vi "GT_EncOn.vi"(2 "encoder":i16, 3 "rtn_In":cluster{"rtn":i16, "Func":string}) -> (0 "encoder out":i16, 1 "rtn_Out":cluster{"rtn":i16, "Func":string})   [LabVIEW 2014]
uses:
  VC6/gts.dll
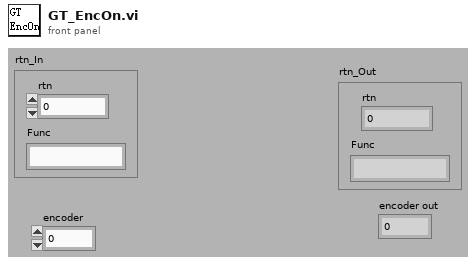
[diagram p1: front panel]
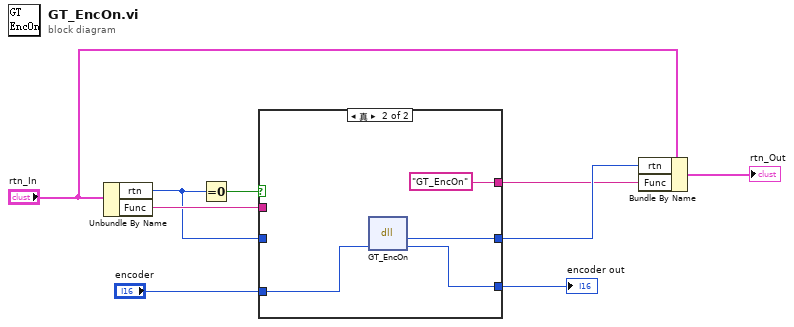
[diagram p0: block diagram]
diagram:
  n1 = Unbundle By Name("rtn_In") -> ("rtn"=w2:i16, "Func"=w8:string)
  n2 = Equal To 0?(x=w2) -> (x = 0?=w9:bool)
  n3 = case shown="真" w9 {
    tunnel: w8 -> [w12 _]
    tunnel: "encoder" -> [w10 w16]
    tunnel: [w11 w15] -> w4
    tunnel: [w12 "GT_EncOn" ("Func")] -> w3
    tunnel: w2 -> [w11 _]
    tunnel: [w10 w13] -> w1
    frame False {
    }
    frame True {
      n4 = dll-call lib="PTH2Fabs DNewGTS AC-800LWin7版源程序-20170926gts85VC6gts.dll" fn="GT_EncOn"("encoder"=w16) -> ("rtn"=w15:i16, "encoder"=w13:i16)  [unwired: 3 in, 2 out]
    }
  }
  "encoder out" <- w1
  n5 = Bundle By Name(cluster="rtn_In", "rtn"=w4, "Func"=w3) -> (→"rtn_Out":cluster{"rtn":i16, "Func":string})
